vi "Damped Oscillator.vi"() -> ()   [LabVIEW 2024]
uses:
  <vilib>/Analysis/2dsp.llb/Real FFT.vi
  <vilib>/express/express analysis/Spectral/Block/exnSpectralBlock spectral measurements RMS poly.vi
  <vilib>/express/express analysis/Spectral/Block/exnSpectralBlock spectral measurements RMS WFM.vi
  <vilib>/express/express analysis/Spectral/XNode/ExpressSpectralMeasurementsBlockNode.xnode
  <vilib>/Analysis/NI_AALPro.lvlib
panel:
  in  "parameters":T1={"Amplitude"=1.0, "Frequency"=440.0, "damping"=10.0}
  out "Complex plane":cluster{dbl[], dbl[]}(graph)
  out "FFT":waveform(dbl)[](graph)=[{"t0"=timestamp(0 s since 1904-01-01), "dt"=1.0, "Y"=array[48000 elements]}, {"t0"=timestamp(0 s since 1904-01-01), "dt"=1.0, "Y"=array[48000 elements]}]
  out "spectrum of damped wave":cluster{"f0":dbl, "df":dbl, "magnitude":dbl[]}(graph)={"f0"=0.0, "df"=1.0, "magnitude"=array[24000 elements]}
  out "damped sine wave":waveform(dbl)(graph)={"t0"=timestamp(0 s since 1904-01-01), "dt"=2.0833333333333333e-05, "Y"=array[48000 elements]}
  out "sine wave":waveform(dbl)(graph)={"t0"=timestamp(0 s since 1904-01-01), "dt"=2.0833333333333333e-05, "Y"=array[48000 elements], "attributes"=variant("NI_ChannelName"=variant(string "Sine"), "NI_ExpIsRelativeTime"=variant(bool TRUE), "NI_ExpStartTimeStamp"=variant(timestamp timestamp(3827639743.002743 s since 1904-01-01)), "NI_ExpTimeStamp"=variant(timestamp timestamp(3827639743.002743 s since 1904-01-01)), "NI_ExpXDimension"=variant(string "t"))}
  out "Spectrum of sine waves":cluster{"f0":dbl, "df":dbl, "magnitude":dbl[]}(graph)={"f0"=0.0, "df"=1.0, "magnitude"=array[24000 elements]}
  # "Parameters"
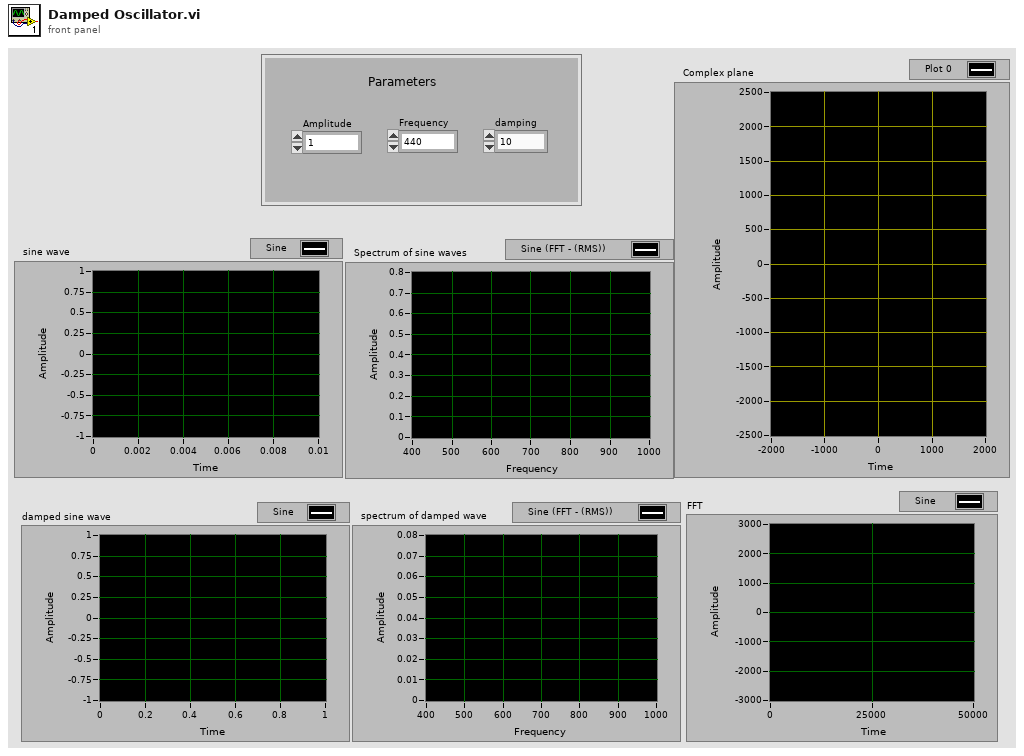
[diagram p1: front panel]
types:
  T1 = cluster{"Amplitude":dbl, "Frequency":dbl, "damping":dbl}
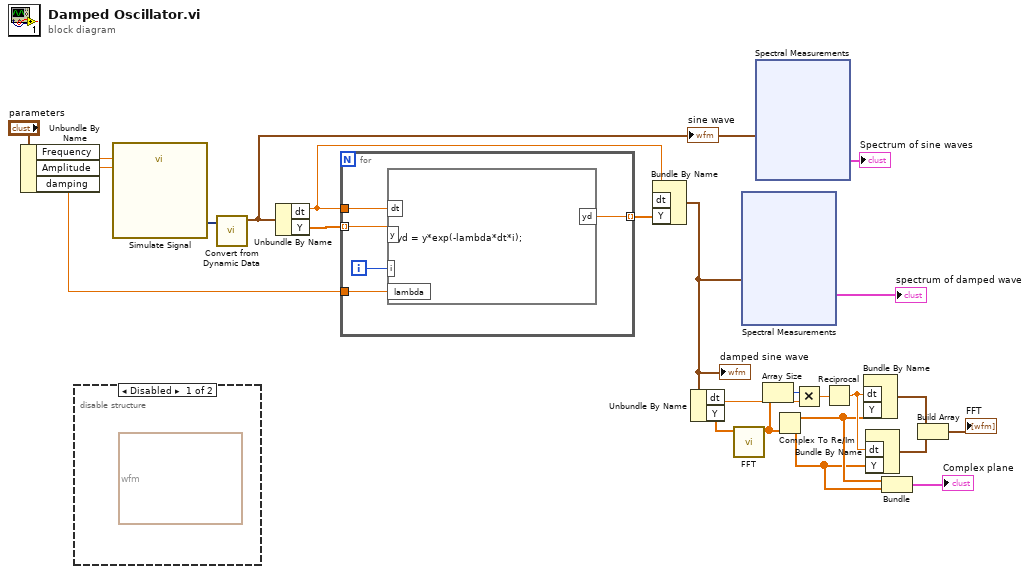
[diagram p0: block diagram]
diagram:
  n1 = Unbundle By Name("parameters") -> ("Frequency"=w3:dbl, "Amplitude"=w2:dbl, "damping"=w1:dbl)
  n2 = disable-structure shown="Disabled" {
    frame Disabled {
      (unwired) waveform(dbl) {"t0"=timestamp(0 s since 1904-01-01), "dt"=2.0833333333333333e-05, "Y"=array[288010 elements]} ("element")
    }
    frame Enabled {
    }
  }
  n3 = call "Simulate Signal"("Frequency"=w3, "Amplitude"=w2) -> ("Sine"=w8:dynamicdata)  [unwired: 12 in, 1 out]
  n4 = call "Convert from Dynamic Data"("Dynamic Data Type"=w8) -> ("Waveform"=w5:waveform(dbl))  [unwired: 3 in]
  "sine wave" <- w5
  n5 = Unbundle By Name(w5) -> ("dt"=w12:dbl, "Y"=w7:dbl[])
  n6 = for {
    tunnel: w7 -> [w29] mode=indexing
    tunnel: w12 -> [w27]
    tunnel: [w26] -> w6 mode=indexing
    tunnel: w1 -> [w25]
    i -> [w28]
    n7 = formula code="yd = y*exp(-lambda*dt*i);"("y"=w29, "dt"=w27, "i"=w28, "lambda"=w25) -> ("yd"=w26:dbl)
  }
  n8 = Bundle By Name("dt"=w12, "Y"=w6) -> (w11:waveform(dbl))  [unwired: 1 in]
  "damped sine wave" <- w11
  n9 = Unbundle By Name(w11) -> ("dt"=w10:dbl, "Y"=w9:dbl[])
  n10 = call-poly <vilib>:"FFT.vi"("X"=w9) -> ("FFT {X}"=w22:cdb[])  [unwired: 9 in, 1 out]
  n11 = xnode "Spectral Measurements"("Signals"=w11) -> ("FFT - (RMS)"=→"spectrum of damped wave":cluster{"f0":dbl, "df":dbl, "magnitude":dbl[]})  [unwired: 1 in, 2 out]
  n12 = xnode "Spectral Measurements"("Signals"=w5) -> ("FFT - (RMS)"=→"Spectrum of sine waves":cluster{"f0":dbl, "df":dbl, "magnitude":dbl[]})  [unwired: 1 in, 2 out]
  n13 = Array Size(array=w22) -> (size(s)=w21:i32)
  n14 = Complex To Re/Im(x + iy=w22) -> (x=w15:dbl[], y=w14:dbl[])
  n15 = Multiply(x=w21, y=w10) -> (x*y=w20:dbl)
  n16 = Reciprocal(x=w20) -> (1/x=w19:dbl)
  n17 = Bundle By Name("dt"=w19, "Y"=w15) -> (w18:waveform(dbl))  [unwired: 1 in]
  n18 = Bundle By Name("dt"=w19, "Y"=w14) -> (w17:waveform(dbl))  [unwired: 1 in]
  n19 = Bundle(w15, w14) -> (→"Complex plane":cluster{dbl[], dbl[]})  [unwired: 1 in]
  n20 = Build Array(w18, w17) -> (→"FFT":waveform(dbl)[])
